vi "Is Empty.vi"(1 "a":refnum<class "Bytestream.lvclass">) -> (0 "empty?":bool)   [LabVIEW 2020, in "NI_Bytestream.lvlib" / "Bytestream.lvclass"]
uses:
  <vilib>/Array/Bytestream/Bytestream.lvclass
  <vilib>/Array/Bytestream/Bytestream.lvclass/Bytestream.ctl
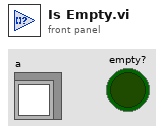
[diagram p1: front panel]
types:
  T1 = typedef "NI_Bytestream.lvlib/Bytestream.lvclass/Datum.ctl" = cluster{"array":u8[], "index":i32}
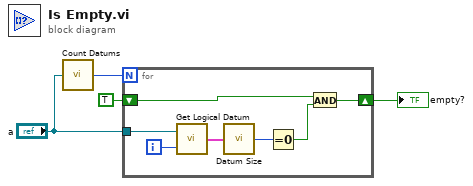
[diagram p0: block diagram]
diagram:
  n1 = call <vilib>:"Count Datums.vi"("bytestream"="a") -> ("datums"=w1:i32)
  n2 = for {
    N: w1 -> [_]
    tunnel: "a" -> [w9]
    shift-right: [w11] -> w3
    shift-left: TRUE -> [w10]
    i -> [w8]
    n3 = call <vilib>:"Get Logical Datum.vi"("index"=w8, "bytestream"=w9) -> ("datum"=w7:T1)
    n4 = call <vilib>:"Datum Size.vi"("datum"=w7) -> ("size"=w6:i32)
    n5 = Equal To 0?(x=w6) -> (x = 0?=w5:bool)
    n6 = And(x=w10, y=w5) -> (x .and. y?=w11:bool)
  }
  "empty?" <- w3
